vi "real time imaging.vi"() -> ()   [LabVIEW 2016]
uses:
  C:/Laser generated ultrasound/Labview/Kinesis Control/Thorlabs.MotionControl.Controls.dll
  Thorlabs.MotionControl.Controls.dll
  C:/Laser generated ultrasound/Labview/Kinesis Control/Thorlabs.MotionControl.KCube.BrushlessMotorCLI.dll
  Thorlabs.MotionControl.KCube.BrushlessMotorCLI.dll
  <vilib>/Analysis/3filter.llb/Filter Passband Type.ctl
  <vilib>/Analysis/baseanly.llb/Mean (DBL).vi
  <vilib>/Analysis/baseanly.llb/Real A x B.vi
  <vilib>/Utility/file.llb/Write To Spreadsheet File (DBL).vi
  <instrlib>/niScope/Acquire/Fetch/niScope Fetch.vi
  <vilib>/Analysis/Matrix/Numeric/Conversions/Array To Matrix - RA2.vi
  <vilib>/Analysis/Matrix/Numeric/Conversions/Matrix To Array - RM.vi
  <vilib>/Analysis/3filter.llb/Butterworth Filter (DBL).vi
  <instrlib>/niScope/Acquire/Fetch/niScope Multi Fetch.vi
  <vilib>/Analysis/NI_AALBase.lvlib
  <vilib>/Analysis/Matrix/NI_Matrix.lvlib
  <vilib>/Analysis/NI_AALPro.lvlib
panel:
  out "Intensity Graph 4":dbl[][](graph)
  out "size(s) 2":i32
  out "Intensity Graph 3":dbl[][](graph)
  out "Intensity Graph 2":dbl[][](graph)
  out "size(s)":i32[](array[numeric])
  in  "stop":bool
  in  "Tab Control":T1(tab)
  in  "File Location":string="C:\\Laser generated ultrasound\\Labview\\Kinesis Control\\test data"
  in  "File name":string="scan_1"
  in  "SerialNumber":string="28251512"
  in  "Scan Length (mm)":dbl=20.0
  in  "Pullback speed (mm/s)":dbl=40.0
  in  "Repetition rate (Hz)":dbl=100.0
  in  "vertical range (V)":dbl=0.5 min=0.0 max=10.0 step=0.5
  in  "Depth (mm)":i32=15
  in  "Start acquisition":bool
  out "Number of samples":dbl
  out "number of a-lines":dbl
  in  "Apply frequency filter":bool
  in  "High Cutoff (MHz)":dbl=45.0
  in  "Low Cutoff (MHz)":dbl=1.0
  in  "Number of points":i32=150
  in  "Exponent":dbl=2.5
  out "?":cluster{dbl[], dbl[]}(graph)
  in  "Preview A-line?":bool
  in  "Start save":bool
  out "Intensity Graph":dbl[][](graph)
  in  "Stop save":bool
  out "Acquiring Data":bool
  out "y":dbl
  in  "KCubeBrushlessControl":refnum<k24>(container)
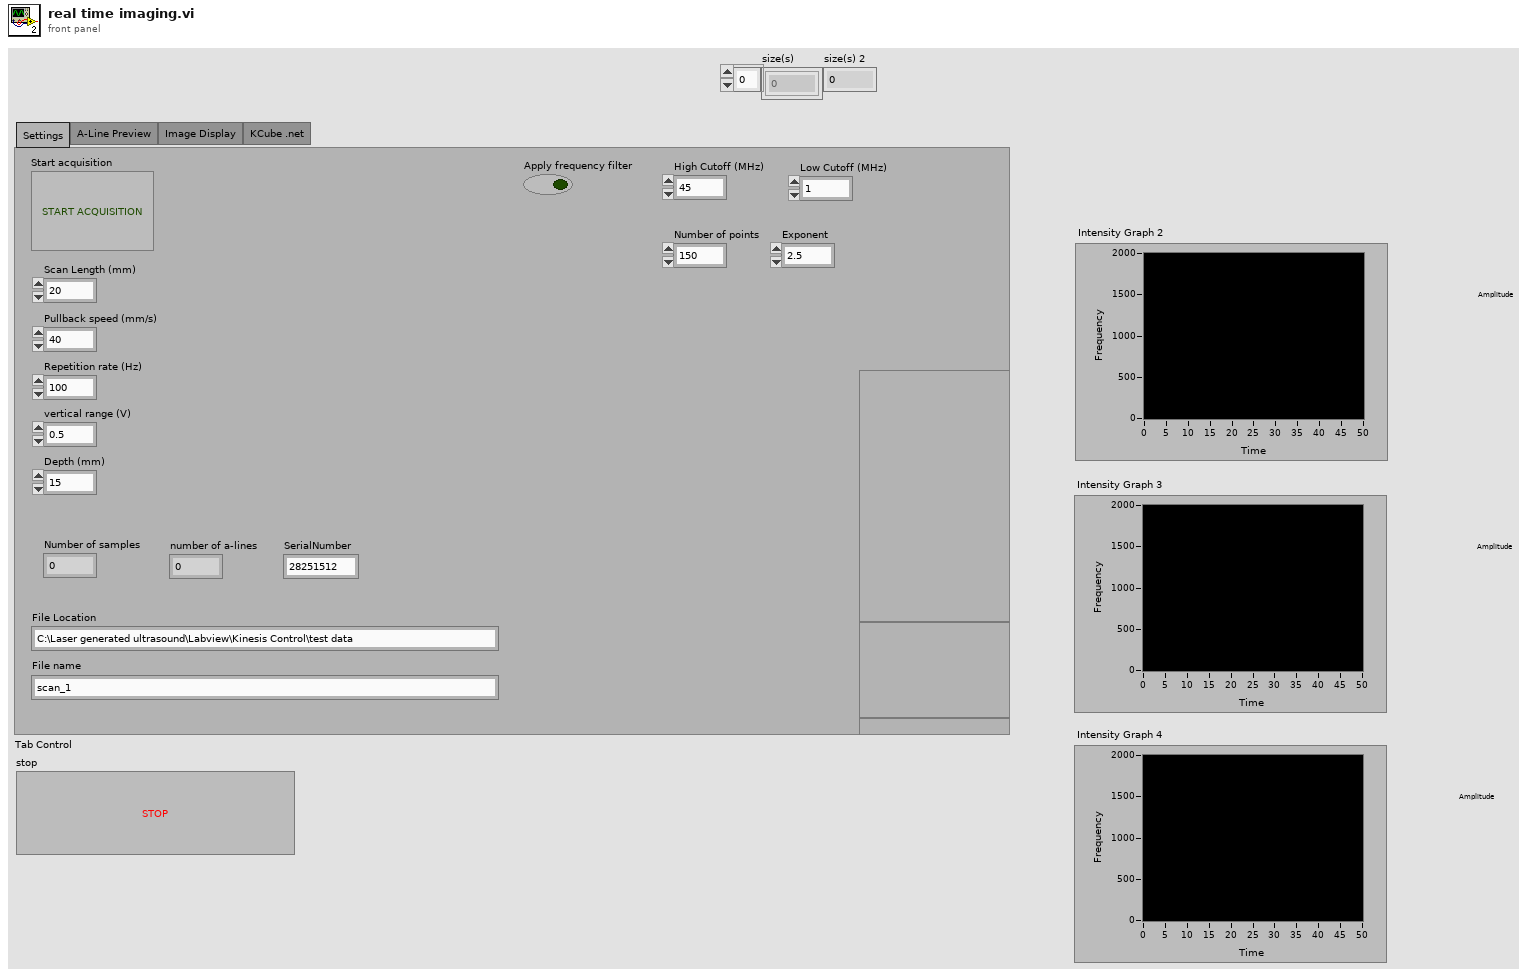
[diagram p1: front panel]
types:
  T1 = enum32{"Settings", "A-Line Preview", "Image Display", "KCube .net"}
  T2 = typedef "NI_AALBase.lvlib/Filter Passband Type.ctl" = enum32{"Lowpass", "Highpass", "Bandpass", "Bandstop"}
  T3 = typedef "NI_Matrix.lvlib/RealMatrix.ctl" = dbl[][]
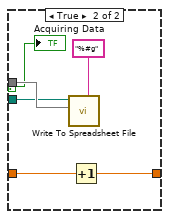
[diagram p8: hidden frame]
diagram:
  n1 = flat-sequence {
    tunnel: [w100] -> w66
    tunnel: [w99] -> w64
    tunnel: [w98] -> w62
    tunnel: [w96] -> w60
    tunnel: [w95] -> w58
    tunnel: [w82] -> w56
    tunnel: [w83] -> w54
    tunnel: ["Scan Length (mm)"] -> w52
    tunnel: ["Pullback speed (mm/s)"] -> w50
    tunnel: [w73] -> w48
    tunnel: ["File Location"] -> w47
    tunnel: ["File name"] -> w46
    tunnel: [w75] -> w38
    tunnel: [w75] -> w35
    tunnel: [w67] -> w5
    tunnel: w66 -> [w160]
    tunnel: [w160] -> w65
    tunnel: w64 -> [w159]
    tunnel: [w159] -> w63
    tunnel: w62 -> [w158]
    tunnel: [w158] -> w61
    tunnel: w60 -> [w157]
    tunnel: [w157] -> w59
    tunnel: w58 -> [w156]
    tunnel: [w156] -> w57
    tunnel: w56 -> [w155]
    tunnel: [w155] -> w55
    tunnel: w54 -> [w154]
    tunnel: [w154] -> w53
    tunnel: w52 -> [w153]
    tunnel: [w153] -> w51
    tunnel: w50 -> [w152]
    tunnel: [w152] -> w49
    tunnel: w48 -> [w150]
    tunnel: w47 -> [w115]
    tunnel: w46 -> [w114]
    tunnel: w38 -> [w122]
    tunnel: [w122] -> w37
    tunnel: w35 -> [w120]
    tunnel: w5 -> [w113]
    tunnel: [w113] -> w4
    tunnel: w65 -> [w173]
    tunnel: w63 -> [w168]
    tunnel: w61 -> [w169]
    tunnel: [w173] -> w45
    tunnel: [w168] -> w44
    tunnel: [w169] -> w43
    tunnel: w59 -> [w167]
    tunnel: w57 -> [w166]
    tunnel: [w167] -> w42
    tunnel: [w166] -> w41
    tunnel: [w165] -> w40
    tunnel: w55 -> [w164]
    tunnel: [w164] -> w39
    tunnel: w53 -> [w165]
    tunnel: w51 -> [_]
    tunnel: w49 -> [w163]
    tunnel: w37 -> [w162]
    tunnel: [w162] -> w36
    tunnel: w4 -> [w161]
    tunnel: [w161] -> w3
    tunnel: w45 -> [w186]
    tunnel: [w186] -> w34
    tunnel: w44 -> [w185]
    tunnel: [w185] -> w32
    tunnel: w43 -> [w184]
    tunnel: [w184] -> w30
    tunnel: w42 -> [w183]
    tunnel: [w182] -> w28
    tunnel: w41 -> [w181]
    tunnel: [w180] -> w26
    tunnel: w40 -> [w179]
    tunnel: [w176] -> w24
    tunnel: w39 -> [w178]
    tunnel: [w175] -> w22
    tunnel: w36 -> [w177]
    tunnel: w3 -> [w174]
    tunnel: [w174] -> w2
    tunnel: w34 -> [w216]
    tunnel: [w216] -> w33
    tunnel: w32 -> [w215]
    tunnel: [w215] -> w31
    tunnel: w30 -> [w214]
    tunnel: [w214] -> w29
    tunnel: w28 -> [w213]
    tunnel: [w213] -> w27
    tunnel: w26 -> [w212]
    tunnel: [w212] -> w25
    tunnel: w24 -> [w211]
    tunnel: [w209] -> w23
    tunnel: w22 -> [w210]
    tunnel: [w208] -> w21
    tunnel: [w204] -> w20
    tunnel: w2 -> [w203]
    tunnel: [w203] -> w1
    tunnel: w33 -> [w228]
    tunnel: w31 -> [w226]
    tunnel: w29 -> [w227]
    tunnel: [w228] -> w19
    tunnel: [w226] -> w17
    tunnel: [w227] -> w15
    tunnel: w27 -> [w225]
    tunnel: w25 -> [w224]
    tunnel: [w225] -> w13
    tunnel: [w224] -> w11
    tunnel: [w220] -> w9
    tunnel: [w219] -> w7
    tunnel: w23 -> [w223]
    tunnel: w21 -> [w222]
    tunnel: w20 -> [w221]
    tunnel: w1 -> [w218]
    tunnel: w19 -> [w484]
    tunnel: [w484] -> w18
    tunnel: w17 -> [w483]
    tunnel: [w483] -> w16
    tunnel: w15 -> [w482]
    tunnel: [w482] -> w14
    tunnel: w13 -> [w481]
    tunnel: [w481] -> w12
    tunnel: w11 -> [w480]
    tunnel: [w480] -> w10
    tunnel: w9 -> [w479]
    tunnel: [w479] -> w8
    tunnel: w7 -> [w478]
    tunnel: [w478] -> w6
    tunnel: w18 -> [w486]
    tunnel: w16 -> [w485]
    tunnel: w14 -> [_]
    tunnel: w12 -> [w490]
    tunnel: w10 -> [w489]
    tunnel: w8 -> [w488]
    tunnel: w6 -> [w487]
    frame #0 {
      # "Initiialise data array"
      # "round trip"
      # "speed of sound"
      # "convert depth to samples"
      # "convert to metre"
      # "Intialise all the equipment\n1. Motor\n2. Trigger\n3. Acquisition"
      n2 = Multiply(x=1500 ("y"), y=1e-08) -> (x*y=w87:dbl)
      n3 = local read "Pullback speed (mm/s)"() -> (w71:dbl)
      n4 = local read "Scan Length (mm)"() -> (w72:dbl)
      n5 = call "pulse_init.vi"("Repetition rate"="Repetition rate (Hz)") -> ("error out"=w95:errorcluster, "Refnum out"=w96:refnum<k21>)  [unwired: 9 in]
      n6 = local read "Repetition rate (Hz)"() -> (w70:dbl)
      n7 = Divide(x="Depth (mm)", y=1000) -> (x/y=w86:dbl)
      n8 = Multiply(x=w86, y=2.0) -> (x*y=w84:dbl)
      n9 = property class="KCubeBrushlessControl"(reference="KCubeBrushlessControl", "SerialNumber"="SerialNumber") -> (reference out=w104:refnum<k24>, error out=w103:errorcluster)  [unwired: 1 in]
      n10 = Divide(x=w84, y=w87) -> (x/y=w90:dbl)
      n11 = Round Toward +Infinity(x=w90) -> (ceil(x): smallest int >= x=w73:dbl)
      "Number of samples" <- w73
      n12 = Initialize Array(0.0 ("element"), w73) -> (w76:dbl[])
      n13 = for {
        N: w73 -> [_]
        shift-right: [w112] -> w75
        shift-left: w76 -> [w111]
        i -> [w110]
        # "Create time axis"
        n14 = To Double Precision Float(number=w110) -> (double precision float=w109:dbl)
        n15 = Multiply(x=w109, y=1e-08) -> (x*y=w107:dbl)
        n16 = Replace Array Subset(array=w111, new element=w107, index=w110) -> (w112:dbl[])
      }
      n17 = Divide(x=w72, y=w71) -> (x/y=w69:dbl)
      n18 = Multiply(x=w69, y=w70) -> (x*y=w68:dbl)
      n19 = call "scope_init.vi"("Num Samples"=w73, "vertical range"="vertical range (V)", "Averages"=1) -> ("error out"=w82:errorcluster, "IVI Refnum out"=w83:refnum<k15>)  [unwired: 7 in]
      n20 = Initialize Array(0.0 ("element"), w73, w68) -> (w67:dbl[][])
      n21 = invoke class="KCubeBrushlessControl" method="CreateDevice"(reference=w104, error in=w103) -> (reference out=w102:refnum<k24>, error out=w101:errorcluster)  [unwired: 1 in, 1 out]
      n22 = property class="KCubeBrushlessControl"(reference=w102, error in=w101) -> (reference out=w100:refnum<k24>, error out=w99:errorcluster, "Device"=w98:refnum<k24>)
    }
    frame #1 {
      w123 = "\r"
      w126 = "\t"
      # "Save the header file"
      # "Initialise the data matrix"
      # "calculate number of a-lines"
      # "Initialise the data matrix\nSave the Header file"
      n23 = local read "Repetition rate (Hz)"() -> (w132:dbl)
      n24 = local read "Number of samples"() -> (w138:dbl)
      n25 = local read "Scan Length (mm)"() -> (w149:dbl)
      n26 = local read "Pullback speed (mm/s)"() -> (w148:dbl)
      n27 = local read "number of a-lines"() -> (w135:dbl)
      n28 = local read "Scan Length (mm)"() -> (w129:dbl)
      n29 = local read "Pullback speed (mm/s)"() -> (w125:dbl)
      n30 = local read "Repetition rate (Hz)"() -> (w146:dbl)
      n31 = Number To Decimal String(number=w138) -> (decimal integer string=w137:string)  [unwired: 1 in]
      n32 = Number To Decimal String(number=w132) -> (decimal integer string=w131:string)  [unwired: 1 in]
      n33 = Number To Decimal String(number=w135) -> (decimal integer string=w134:string)  [unwired: 1 in]
      n34 = Number To Decimal String(number=w129) -> (decimal integer string=w128:string)  [unwired: 1 in]
      n35 = Concatenate Strings(w115, "\\" ("string"), w114, "_hdr.txt" ("string")) -> (w143:string)
      n36 = Divide(x=w149, y=w148) -> (x/y=w147:dbl)
      n37 = Number To Decimal String(number=w125) -> (decimal integer string=w124:string)  [unwired: 1 in]
      n38 = Concatenate Strings(w115, "\\" ("string"), w114, "_taxis.txt" ("string")) -> (w119:string)
      n39 = Multiply(x=w147, y=w146) -> (x*y=w145:dbl)
      "number of a-lines" <- w145
      n40 = String To Path(string=w119) -> (path=w116:path)
      n41 = Initialize Array(0.0 ("element"), w150, w145) -> ()  [unwired: 1 out]
      n42 = call-poly <vilib>:"Write To Spreadsheet File.vi"("format (%.3f)"="%#g", "1D data"=w120, "file path (dialog if empty)"=w116) -> ()  [unwired: 5 in, 1 out]
      n43 = Concatenate Strings("Samples per A-line" ("string"), w126, w137, w123, "Number of A-lines" ("string"), w126, w134, w123, "Repetition rate (Hz)" ("string"), w126, w131, w123, "Scan length (mm)" ("string"), w126, w128, w123, "Pullback speed (mm/s)" ("string"), w126, w124, w123) -> (w140:string)
      n44 = String To Path(string=w143) -> (path=w144:path)
      n45 = Write to Text File(file (use dialog)=w144, text=w140) -> ()  [unwired: 2 in, 3 out]
    }
    frame #2 {
      # "Initial data array"
      # "Home the motor"
      n46 = invoke class="KCubeBrushlessMotor" method="Home"(reference=w169, error in=w168, "waitTimeout"=50000) -> ()  [unwired: 1 in, 4 out]
      n47 = invoke class="KCubeBrushlessMotor" method="SetVelocityParams"(reference=w169, error in=w168, "maxVelocity"=w163, "acceleration"=999.7) -> ()  [unwired: 1 in, 5 out]
      n48 = Wait (ms)(milliseconds to wait=u32 1000) -> ()  [unwired: 1 out]
    }
    frame #3 {
      # "A-line display for positioning"
      n49 = while {
        tunnel: w183 -> [w201]
        tunnel: w181 -> [w200]
        tunnel: [w201] -> w182
        tunnel: [w200] -> w180
        tunnel: w179 -> [w197]
        tunnel: w178 -> [w196]
        tunnel: w177 -> [w191]
        tunnel: [w188] -> w176
        tunnel: [w187] -> w175
        stop <- "Start acquisition" stop-if-true
        n50 = local read "Number of samples"() -> (w199:dbl)
        n51 = call <instrlib>:"niScope Initiate Acquisition.vi"("instrument handle"=w197, "error in"=w196) -> ("instrument handle out"=w195:refnum<k15>, "error out"=w194:errorcluster)  [unwired: 12 in]
        n52 = call-poly <instrlib>:"niScope Fetch (poly).vi"("error in"=w194, "numSamples"=w199, "channels"="0", "instrument handle"=w195) -> ("error out"=w187:errorcluster, "wfm"=w193:dbl[], "instrument handle out"=w188:refnum<k15>)  [unwired: 4 in, 1 out]
        n53 = Bundle(w191, "wfm"=w193) -> (w192:cluster{dbl[], "wfm":dbl[]})  [unwired: 1 in]
        n54 = case shown="True" "Preview A-line?" {
          tunnel: w192 -> [_ w202]
          frame False {
          }
          frame True {
            "?" <- w202
          }
        }
      }
    }
    frame #4 {
      # "Setup acquisition cards to record all a-lines"
      n55 = local read "Number of samples"() -> (w204:dbl)
      n56 = local read "number of a-lines"() -> (w205:dbl)
      n57 = call <instrlib>:"niScope Configure Horizontal Timing.vi"("instrument handle"=w211, "number of records"=w205, "min sample rate"=100000000.0, "reference position"=0.0, "error in"=w210, "min record length"=w204) -> ("instrument handle out"=w209:refnum<k15>, "error out"=w208:errorcluster)  [unwired: 8 in]
    }
    frame #5 {
      w217 = 0.0 ("y")
      # "move to end and acquire data\n1. move motor\n2. acquire data"
      n58 = while {
        tunnel: w227 -> [w257]
        tunnel: w226 -> [w256]
        tunnel: w221 -> [w253]
        shift-right: [w243] -> w220
        shift-left: w223 -> [w255]
        shift-right: [w242] -> w219
        shift-left: w222 -> [w254]
        shift-right: [w240] -> _
        shift-left: w218 -> [w239]
        shift-right: [w238] -> _
        shift-left: w217 -> [w236]
        shift-right: [w234] -> _
        shift-left: w217 -> [w233]
        shift-right: [w231] -> _
        shift-left: w217 -> [w230]
        stop <- "stop" stop-if-true
        # "Image number increment"
        # "Numeric to act as boolean to keep save going"
        n59 = call <instrlib>:"niScope Initiate Acquisition.vi"("instrument handle"=w255, "error in"=w254) -> ("instrument handle out"=w252:refnum<k15>, "error out"=w251:errorcluster)  [unwired: 12 in]
        n60 = flat-sequence {
          tunnel: w257 -> [w312]
          tunnel: w256 -> [w311]
          tunnel: w253 -> [w310]
          tunnel: w252 -> [w306]
          tunnel: w251 -> [w305]
          tunnel: [w309] -> w250
          tunnel: [w308] -> w249
          tunnel: [w275] -> w248
          tunnel: [w275] -> w247
          tunnel: [w301] -> w245
          tunnel: [w300] -> w244
          tunnel: w239 -> [w263]
          tunnel: [w297] -> w241
          tunnel: [w291] -> w237
          tunnel: w236 -> [w289]
          tunnel: w233 -> [w284]
          tunnel: [w283] -> w235
          tunnel: w230 -> [w282]
          tunnel: [w282] -> w232
          tunnel: ["Apply frequency filter"] -> w229
          tunnel: [w407] -> w242
          tunnel: [w408] -> w243
          tunnel: w250 -> [w410]
          tunnel: w249 -> [w409]
          tunnel: w248 -> [w413]
          tunnel: w247 -> [w372]
          tunnel: w245 -> [w406]
          tunnel: w244 -> [w405]
          tunnel: w241 -> [w400]
          tunnel: [w399] -> w240
          tunnel: [w398] -> w238
          tunnel: w237 -> [w392]
          tunnel: w235 -> [w382]
          tunnel: [w396] -> w234
          tunnel: w232 -> [w391]
          tunnel: [w393] -> w231
          tunnel: w229 -> [w369]
          frame #0 {
            w266 = 20 ("length")
            # "Frequency filter"
            # "cross-talk removal"
            # "Calculate the running average"
            # "take first few A-lines to repeat and use for running average"
            # "0 - 2000 - time\n1 - 50 - a-lines"
            # "NEXT STEPS:\nADD in crosstalk removal etc.\n\nWork on the timing for motor movements"
            n61 = local read "Scan Length (mm)"() -> (w302:dbl)
            n62 = local read "Number of samples"() -> (w267:dbl)
            n63 = Number To Decimal String(number=w282) -> (decimal integer string=w281:string)  [unwired: 1 in]
            n64 = Number To Decimal String(number=w289) -> (decimal integer string=w279:string)  [unwired: 1 in]
            n65 = Array Size(array=w263) -> (size(s)=→"size(s)":i32[])
            n66 = local read "File Location"() -> (w294:string)
            n67 = local read "File name"() -> (w292:string)
            n68 = invoke class="KCubeBrushlessMotor" method="MoveTo"(reference=w312, error in=w311, "position"=w302, "waitTimeout"=0) -> (reference out=w301:refnum<k24>, error out=w300:errorcluster)  [unwired: 1 in, 3 out]
            n69 = Array Subset(array=w263, index (row)=0 ("index"), length (row)=w267, index (col)=0 ("index"), length (col)=w266) -> (w270:dbl[][])
            n70 = Concatenate Strings(w294, "\\" ("string"), w292, "_image_" ("string"), w281, "_f_" ("string"), w279, ".txt" ("string")) -> (w296:string)
            n71 = for {
              tunnel: w270 -> [w358] mode=indexing
              tunnel: [w357] -> w269 mode=indexing
              n72 = Reverse 1D Array(array=w358) -> (reversed array=w357:dbl[])
            }
            n73 = call-poly <instrlib>:"niScope Fetch (poly).vi"("timeout"=-1.0, "error in"=w305, "numSamples"=w310, "channels"="0", "instrument handle"=w306) -> ("error out"=w308:errorcluster, "wfm"=w276:dbl[][], "instrument handle out"=w309:refnum<k15>)  [unwired: 3 in, 1 out]
            n74 = String To Path(string=w296) -> (path=w295:path)
            n75 = Equal?(x=w284, y=1.0) -> (x = y?=w286:bool)
            n76 = Or(x="Start save", y=w286) -> (x .or. y?=w288:bool)
            n77 = local read "number of a-lines"() -> (w265:dbl)
            n78 = Insert Into Array(array=w263, index (col)=0 ("disabled index (col)"), new element=w269) -> (w268:dbl[][])  [unwired: 1 in]
            n79 = case shown="True" w288 {
              tunnel: w263 -> [_ w364]
              tunnel: w295 -> [_ w363]
              tunnel: [w361 w362] -> w291
              tunnel: w289 -> [w361 w362]
              frame False {
              }
              frame True {
                n80 = call-poly <vilib>:"Write To Spreadsheet File.vi"("format (%.3f)"="%#g", "2D data"=w364, "file path (dialog if empty)"=w363) -> ()  [unwired: 5 in, 1 out]
              }
            }
            n81 = for {
              N: w265 -> [_]
              tunnel: w268 -> [w354]
              tunnel: w267 -> [w352]
              tunnel: w266 -> [w350]
              tunnel: [w348] -> w264 mode=indexing
              i -> [w351]
              n82 = Array Subset(array=w354, index (row)=0 ("index"), length (row)=w352, index (col)=w351, length (col)=w350) -> (w349:dbl[][])
              n83 = for {
                tunnel: w349 -> [w356] mode=indexing
                tunnel: [w355] -> w348 mode=indexing
                n84 = call-poly <vilib>:"Mean.vi"("X"=w356) -> ("mean"=w355:dbl)  [unwired: 1 out]
              }
            }
            "Intensity Graph 2" <- w264
            n85 = Transpose 2D Array(2D array=w276) -> (transposed array=w275:dbl[][])
            n86 = case shown="True" "Start save" {
              tunnel: w284 -> [w359 _]
              tunnel: [w359 1.0 ("y")] -> w283
              frame False {
              }
              frame True {
              }
            }
            n87 = Transpose 2D Array(2D array=w263) -> (transposed array=w262:dbl[][])
            "Intensity Graph 3" <- w262
            n88 = Replace Array Subset(array=w263, new element=w275, index (row)=0, index (col)=0 ("disabled index (col)")) -> (w297:dbl[][])
            n89 = for {
              N: w265 -> [_]
              tunnel: w264 -> [w341] mode=indexing
              tunnel: w262 -> [w340] mode=indexing
              tunnel: [w338] -> w261 mode=indexing
              n90 = call "create_design_matrix.vi"("input vector"=w341) -> ("design matrix"=w347:dbl[][])
              n91 = Array Size(array=w340) -> (size(s)=w342:i32)
              "size(s) 2" <- w342
              n92 = call "linear_fit.vi"("Real 1D Array"=w340, "X"=w347) -> ("A x B"=w346:T3)
              n93 = call-poly <vilib>:"Array To Matrix.vi"("Real 2D Array"=w347) -> ("Real Matrix"=w345:T3)
              n94 = call-poly <vilib>:"A x B.vi"("B"=w345, "A"=w346) -> ("A x B"=w344:T3)  [unwired: 1 out]
              n95 = call-poly <vilib>:"Matrix To Array.vi"("Real Matrix"=w344) -> ("Real 2D Array"=w343:dbl[][])
              n96 = Reshape Array(w343, w342) -> (w339:dbl[])
              n97 = Subtract(x=w340, y=w339) -> (x-y=w338:dbl[])
            }
            n98 = Wait (ms)(milliseconds to wait=u32 1000) -> ()  [unwired: 1 out]
            n99 = case shown="True" "Apply frequency filter" {
              tunnel: w261 -> [w320 w322]
              tunnel: [w320 w321] -> w260
              frame False {
              }
              frame True {
                n100 = Multiply(x="High Cutoff (MHz)", y=1000000.0) -> (x*y=w328:dbl)
                n101 = Multiply(x="Low Cutoff (MHz)", y=1000000.0) -> (x*y=w327:dbl)
                n102 = for {
                  tunnel: 100000000.0 ("y") -> [w334]
                  tunnel: w328 -> [w333]
                  tunnel: w327 -> [w332]
                  tunnel: w322 -> [w331] mode=indexing
                  tunnel: [w330] -> w321 mode=indexing
                  n103 = call-poly <vilib>:"Butterworth Filter.vi"("init/cont (init:F)"=FALSE, "order"=8, "filter type"=Filter_Passband_Type."Bandpass", "low cutoff freq: fl"=w332, "high cutoff freq: fh"=w333, "sampling freq: fs"=w334, "X"=w331) -> ("Filtered X"=w330:dbl[])  [unwired: 1 in, 1 out]
                }
              }
            }
            n104 = for {
              tunnel: w260 -> [w319] mode=indexing
              tunnel: [w313] -> w259 mode=indexing
              n105 = call <vilib>:"Fast Hilbert Transform.vi"("X"=w319) -> ("Hilbert{X}"=w318:dbl[])  [unwired: 1 out]
              n106 = Absolute Value(x=w318) -> (abs(x)=w317:dbl[])
              n107 = call "TGC_exponential.vi"("Exponent"="Exponent", "Number of points"="Number of points", "Input vector"=w317) -> ("Output vector"=w314:dbl[])
              n108 = Logarithm Base 10(1:w314) -> (0:w313:dbl[])
            }
            "Intensity Graph" <- w259
            "Intensity Graph 4" <- w259
            "y" <- w284
          }
          frame #1 {
            w377 = 20 ("length")
            # "Frequency filter"
            # "cross-talk removal"
            # "Calculate the running average"
            n109 = local read "File name"() -> (w414:string)
            n110 = local read "File Location"() -> (w415:string)
            n111 = Number To Decimal String(number=w391) -> (decimal integer string=w389:string)  [unwired: 1 in]
            n112 = Number To Decimal String(number=w392) -> (decimal integer string=w387:string)  [unwired: 1 in]
            n113 = invoke class="KCubeBrushlessMotor" method="MoveTo"(reference=w406, error in=w405, "position"=0.0, "waitTimeout"=0) -> ()  [unwired: 1 in, 5 out]
            n114 = Concatenate Strings(w415, "\\" ("string"), w414, "_image_" ("string"), w389, "_b_" ("string"), w387, ".txt" ("string")) -> (w418:string)
            n115 = local read "Number of samples"() -> (w376:dbl)
            n116 = String To Path(string=w418) -> (path=w416:path)
            n117 = call-poly <instrlib>:"niScope Fetch (poly).vi"("timeout"=-1.0, "error in"=w409, "channels"="0", "instrument handle"=w410) -> ("error out"=w407:errorcluster, "wfm"=w384:dbl[][], "instrument handle out"=w408:refnum<k15>)  [unwired: 4 in, 1 out]
            n118 = Equal?(x=1.0, y=w382) -> (x = y?=w395:bool)
            n119 = case shown="False" w395 {
              selector: w395 -> [w470 w472]
              tunnel: w413 -> [_ w476]
              tunnel: w416 -> [_ w475]
              tunnel: w392 -> [_ w474]
              tunnel: [0.0 w473] -> w398
              frame False {
                n120 = local write "Acquiring Data"(w470) -> ()
              }
              frame True {
                n121 = call-poly <vilib>:"Write To Spreadsheet File.vi"("format (%.3f)"="%#g", "2D data"=w476, "file path (dialog if empty)"=w475) -> ()  [unwired: 5 in, 1 out]
                n122 = Increment(x=w474) -> (x+1=w473:dbl)
                "Acquiring Data" <- w472
              }
            }
            n123 = Array Subset(array=w372, index (row)=0 ("index"), length (row)=w376, index (col)=0 ("index"), length (col)=w377) -> (w375:dbl[][])
            n124 = Transpose 2D Array(2D array=w384) -> (transposed array=w383:dbl[][])
            n125 = for {
              tunnel: w375 -> [w455] mode=indexing
              tunnel: [w454] -> w374 mode=indexing
              n126 = Reverse 1D Array(array=w455) -> (reversed array=w454:dbl[])
            }
            n127 = local read "number of a-lines"() -> (w366:dbl)
            n128 = Wait (ms)(milliseconds to wait=u32 1000) -> ()  [unwired: 1 out]
            n129 = Insert Into Array(array=w372, index (col)=0 ("disabled index (col)"), new element=w374) -> (w378:dbl[][])  [unwired: 1 in]
            n130 = for {
              N: w366 -> [_]
              tunnel: w378 -> [w462]
              tunnel: w376 -> [w460]
              tunnel: w377 -> [w458]
              tunnel: [w456] -> w373 mode=indexing
              i -> [w459]
              n131 = Array Subset(array=w462, index (row)=0 ("index"), length (row)=w460, index (col)=w459, length (col)=w458) -> (w457:dbl[][])
              n132 = for {
                tunnel: w457 -> [w464] mode=indexing
                tunnel: [w463] -> w456 mode=indexing
                n133 = call-poly <vilib>:"Mean.vi"("X"=w464) -> ("mean"=w463:dbl)  [unwired: 1 out]
              }
            }
            n134 = case shown="True" "Stop save" {
              tunnel: w382 -> [w466 _]
              tunnel: [w466 0.0 ("y")] -> w396
              tunnel: w391 -> [w465 w468]
              tunnel: [w465 w467] -> w393
              frame False {
              }
              frame True {
                n135 = Increment(x=w468) -> (x+1=w467:dbl)
              }
            }
            n136 = Replace Array Subset(array=w400, new element=w383, index (row)=0, index (col)=0 ("disabled index (col)")) -> (w399:dbl[][])
            n137 = Transpose 2D Array(2D array=w372) -> (transposed array=w371:dbl[][])
            n138 = for {
              N: w366 -> [_]
              tunnel: w373 -> [w447] mode=indexing
              tunnel: w371 -> [w446] mode=indexing
              tunnel: [w444] -> w370 mode=indexing
              n139 = call "create_design_matrix.vi"("input vector"=w447) -> ("design matrix"=w453:dbl[][])
              n140 = Array Size(array=w446) -> (size(s)=w448:i32)
              n141 = call "linear_fit.vi"("Real 1D Array"=w446, "X"=w453) -> ("A x B"=w452:T3)
              n142 = call-poly <vilib>:"Array To Matrix.vi"("Real 2D Array"=w453) -> ("Real Matrix"=w451:T3)
              n143 = call-poly <vilib>:"A x B.vi"("B"=w451, "A"=w452) -> ("A x B"=w450:T3)  [unwired: 1 out]
              n144 = call-poly <vilib>:"Matrix To Array.vi"("Real Matrix"=w450) -> ("Real 2D Array"=w449:dbl[][])
              n145 = Reshape Array(w449, w448) -> (w445:dbl[])
              n146 = Subtract(x=w446, y=w445) -> (x-y=w444:dbl[])
            }
            n147 = case shown="True" w369 {
              tunnel: w370 -> [w426 w430]
              tunnel: [w426 w429] -> w368
              frame False {
              }
              frame True {
                n148 = local read "High Cutoff (MHz)"() -> (w428:dbl)
                n149 = local read "Low Cutoff (MHz)"() -> (w427:dbl)
                n150 = Multiply(x=w428, y=1000000.0) -> (x*y=w434:dbl)
                n151 = Multiply(x=w427, y=1000000.0) -> (x*y=w433:dbl)
                n152 = for {
                  tunnel: 100000000.0 ("y") -> [w440]
                  tunnel: w434 -> [w439]
                  tunnel: w433 -> [w438]
                  tunnel: w430 -> [w437] mode=indexing
                  tunnel: [w436] -> w429 mode=indexing
                  n153 = call-poly <vilib>:"Butterworth Filter.vi"("init/cont (init:F)"=FALSE, "order"=8, "filter type"=Filter_Passband_Type."Bandpass", "low cutoff freq: fl"=w438, "high cutoff freq: fh"=w439, "sampling freq: fs"=w440, "X"=w437) -> ("Filtered X"=w436:dbl[])  [unwired: 1 in, 1 out]
                }
              }
            }
            n154 = for {
              tunnel: w368 -> [w425] mode=indexing
              tunnel: [w421] -> w367 mode=indexing
              n155 = local read "Number of points"() -> (w420:i32)
              n156 = call <vilib>:"Fast Hilbert Transform.vi"("X"=w425) -> ("Hilbert{X}"=w424:dbl[])  [unwired: 1 out]
              n157 = local read "Exponent"() -> (w419:dbl)
              n158 = Absolute Value(x=w424) -> (abs(x)=w423:dbl[])
              n159 = call "TGC_exponential.vi"("Exponent"=w419, "Number of points"=w420, "Input vector"=w423) -> ("Output vector"=w422:dbl[])
              n160 = Logarithm Base 10(1:w422) -> (0:w421:dbl[])
            }
            n161 = local write "Intensity Graph"(w367) -> ()
          }
        }
      }
    }
    frame #6 {
      # "Save data"
    }
    frame #7 {
      # "Close everything"
      n162 = call <vilib>:"DAQmx Stop Task.vi"("task/channels in"=w490, "error in"=w489) -> ("task out"=w492:refnum<k21>, "error out"=w491:errorcluster)  [unwired: 12 in]
      n163 = call <instrlib>:"niScope Close.vi"("instrument handle"=w488, "error in"=w487) -> ()  [unwired: 13 in, 1 out]
      n164 = call <vilib>:"DAQmx Clear Task.vi"("task in"=w492, "error in"=w491) -> ()  [unwired: 13 in, 1 out]
      n165 = invoke class="KCubeBrushlessControl" method="CloseDevice"(reference=w486, error in=w485) -> ()  [unwired: 1 in, 3 out]
    }
  }
